vi "InvMC-Multiplication.vi"(11 "Vector In":u8[](array[numeric]) format="%.0x") -> (3 "Vector Out":u8[](array[numeric]) format="%.0x")   [LabVIEW 2010, in "Encryption.lvlib"]
doc: "Perfroms the Inv MC multiplication lookup for AES.\n\n(c) Ton Plomp, 2011\nTHIS SOFTWARE IS PROVIDED AS IS, AND ANY WARRANTY IS REJECTED"
uses:
  Encryption.lvlib
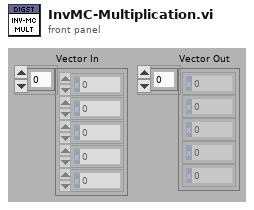
[diagram p1: front panel]
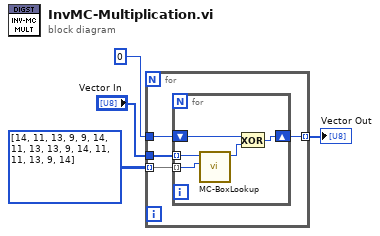
[diagram p0: block diagram]
diagram:
  n1 = for {
    tunnel: "Vector In" -> [w8]
    tunnel: u8[][] [[14, 11, 13, 9], [9, 14, 11, 13], [13, 9, 14, 11], [11, 13, 9, 14]] ("transposed array") -> [w7] mode=indexing
    tunnel: [w6] -> w2 mode=indexing
    tunnel: u8 0 -> [w5]
    n2 = for {
      tunnel: w8 -> [w13] mode=indexing
      tunnel: w7 -> [w12] mode=indexing
      shift-right: [w9] -> w6
      shift-left: w5 -> [w11]
      n3 = call "MC-BoxLookup.vi"("Multiplication"=w12, "Value-In"=w13) -> ("LookUp-Out"=w10:u8)  [unwired: 9 in]
      n4 = Exclusive Or(1:w10, 2:w11) -> (0:w9:u8)
    }
  }
  "Vector Out" <- w2
